vi "find com.vi"() -> (0 "连接了开发板？":bool=TRUE, 1 "VISA resource name out":refnum<visa-resource-name>)   [LabVIEW 2012]
uses:
  <vilib>/Instr/_visa.llb/VISA Flush IO Buffer Mask.ctl
  <vilib>/Instr/_visa.llb/VISA Configure Serial Port (Instr).vi
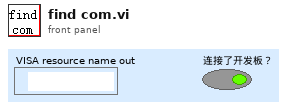
[diagram p1: front panel]
types:
  T1 = typedef "VISA Flush IO Buffer Mask.ctl" = u16
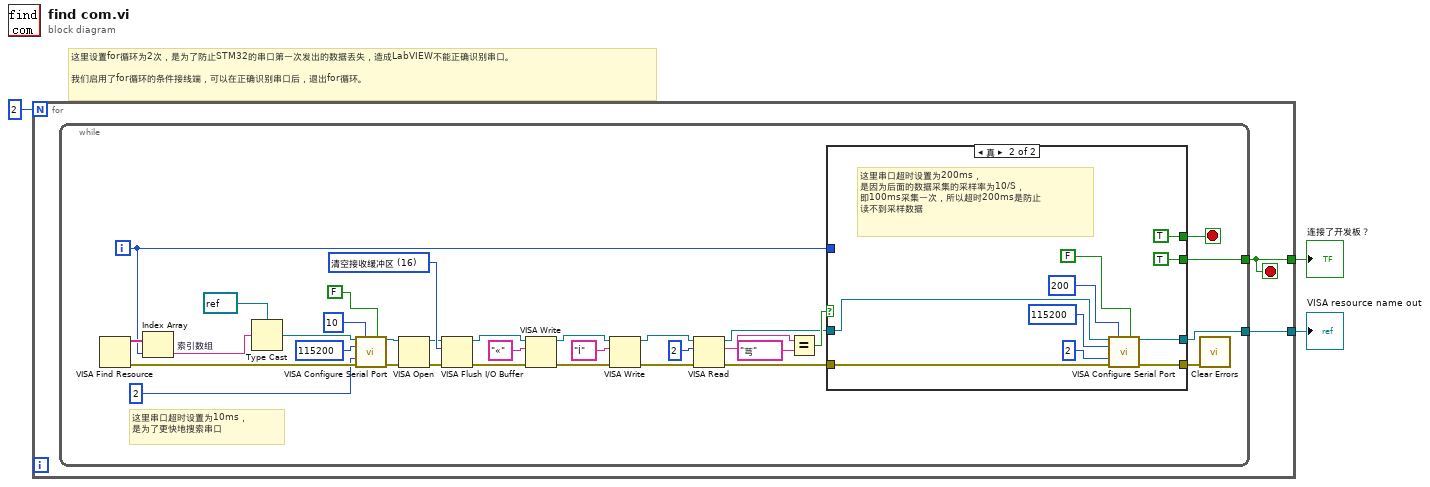
[diagram p0: block diagram]
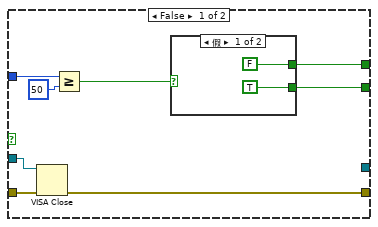
[diagram p2: hidden frame]
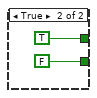
[diagram p3: hidden frame]
diagram:
  # "这里设置for循环为2次，是为了防止STM32的串口第一次发出的数据丢失，造成LabVIEW不能正确识别串口。\n\n我们启用了for循环的条件接线端，可以在正确识别串口后，退出for循环。"
  n1 = for {
    N: 2 -> [_]
    tunnel: [w5] -> w3
    tunnel: [w4] -> w2
    stop <- w4 stop-if-true
    n2 = while {
      tunnel: [w26] -> w5
      tunnel: [w19] -> w4
      i -> [w30]
      stop <- w29 stop-if-true
      w20 = T1 16 items=["清空接收缓冲区"=16, "向设备写入传输缓冲区"=32, "清空接收缓冲区（无I/O）"=64, "清空传输缓冲区"=128] ("Mask")
      # "这里串口超时设置为10ms，\n是为了更快地搜索串口"
      n3 = VISA Find Resource() -> (0:w28:errorcluster, 3:w38:string[])  [unwired: 1 in, 3 out]
      n4 = Index Array "索引数组"(array=w38, index=w30) -> (element=w31:string)
      n5 = Type Cast(type=refnum<visa-resource-name> refnum, x=w31) -> (*(type *) &x=w37:refnum<visa-resource-name>)
      n6 = call-poly "VISA Configure Serial Port"("VISA resource name"=w37, "timeout (10sec)"=u32 10, "Enable Termination\nChar (T)"=FALSE ("Enable Termination\nChar (T)"), "baud rate (9600)"=u32 115200 ("baud rate (460800)"), "parity (0:none)"=u32 2 ("timeout (10sec)"), "error in (no error)"=w28) -> ("VISA resource name out"=w17:refnum<visa-resource-name>, "error out"=w15:errorcluster)  [unwired: 2 in, 6 out]
      n7 = VISA Open(error in (no error)=w15, VISA resource name=w17) -> (VISA resource name=w16:refnum<visa-resource-name>, error out=w14:errorcluster)  [unwired: 3 out]
      n8 = VISA Flush I/O Buffer(VISA resource name=w16, mask (16)=w20, error in (no error)=w14) -> (VISA resource name out=w18:refnum<visa-resource-name>, error out=w24:errorcluster)
      n9 = VISA Write(VISA resource name=w18, write buffer="«", error in (no error)=w24) -> (VISA resource name out=w10:refnum<visa-resource-name>, error out=w8:errorcluster)  [unwired: 1 out]
      n10 = VISA Write(VISA resource name=w10, write buffer="Í", error in (no error)=w8) -> (VISA resource name out=w9:refnum<visa-resource-name>, error out=w7:errorcluster)  [unwired: 1 out]
      n11 = VISA Read(VISA resource name=w9, byte count=u32 2, error in (no error)=w7) -> (VISA resource name out=w27:refnum<visa-resource-name>, read buffer=w32:string, error out=w13:errorcluster)  [unwired: 1 out]
      n12 = Equal?(x=w32, y="芎") -> (x = y?=w34:bool)
      n13 = case shown="真" w34 {
        tunnel: [w43 TRUE] -> w29
        tunnel: w30 -> [w46 _]
        tunnel: w27 -> [w42 w58]
        tunnel: [_ w54] -> w26
        tunnel: [w41 TRUE] -> w19
        tunnel: w13 -> [w40 w53]
        tunnel: [w39 w52] -> w12
        frame False {
          n14 = VISA Close(VISA resource name=w42, error in (no error)=w40) -> (error out=w39:errorcluster)
          n15 = Greater Or Equal?(x=w46, y=50) -> (x >= y?=w44:bool)
          n16 = case shown="假" w44 {
            tunnel: [FALSE TRUE] -> w43
            tunnel: [TRUE FALSE] -> w41
            frame False {
            }
            frame True {
            }
          }
        }
        frame True {
          # "这里串口超时设置为200ms，\n是因为后面的数据采集的采样率为10/S，\n即100ms采集一次，所以超时200ms是防止\n读不到采样数据"
          n17 = call-poly "VISA Configure Serial Port"("VISA resource name"=w58, "timeout (10sec)"=u32 200, "Enable Termination\nChar (T)"=FALSE ("Enable Termination\nChar (T)"), "baud rate (9600)"=u32 115200, "parity (0:none)"=u32 2 ("timeout (10sec)"), "error in (no error)"=w53) -> ("VISA resource name out"=w54:refnum<visa-resource-name>, "error out"=w52:errorcluster)  [unwired: 2 in, 6 out]
        }
      }
      n18 = call <vilib>:"Clear Errors.vi"("error in (no error)"=w12) -> ()  [unwired: 6 in, 1 out]
    }
  }
  "VISA resource name out" <- w3
  "连接了开发板？" <- w2
